vi "Open PolarizationProcessorSDK.vi"(8 "error in (no error)":errorcluster) -> (0 "error out":errorcluster, 3 "PolarizationProcessorSDK reference":refnum<k24>)   [LabVIEW 2015]
uses:
  C:/code/Host/Installer/Scientific Camera Interfaces/LabVIEW/32_bit/Library_X86/Thorlabs.TSI.PolarizationProcessor.dll
  code/Host/Installer/Scientific Camera Interfaces/LabVIEW/32_bit/Library_X86/Thorlabs.TSI.PolarizationProcessor.dll
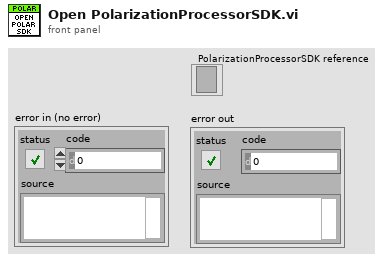
[diagram p1: front panel]
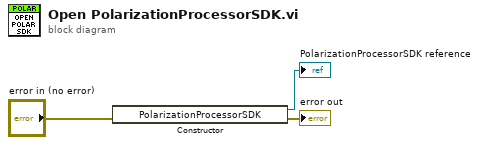
[diagram p0: block diagram]
diagram:
  n1 = constructor class="PolarizationProcessorSDK"(error in="error in (no error)") -> (reference out=→"PolarizationProcessorSDK reference":refnum<k24>, error out=→"error out":errorcluster)  [unwired: 2 in, 1 out]
